vi "Query Client for Token.vi"(8 "error in (no error)":errorcluster, 10 "Request URI":string, 11 "OAuthClient in":refnum<class "OAuthClient.lvclass">) -> (0 "error out":errorcluster, 1 "Body":string, 2 "Header":string, 3 "OAuthClient out":refnum<class "OAuthClient.lvclass">)   [LabVIEW 2013, in "OAuthClient.lvclass"]
uses:
  OAuthClient.lvclass
  OAuthClient.lvclass/OAuthClient.ctl
  <vilib>/httpClient/POSTBuffer.vi
  <vilib>/httpClient/LabVIEWHTTPClient.lvlib
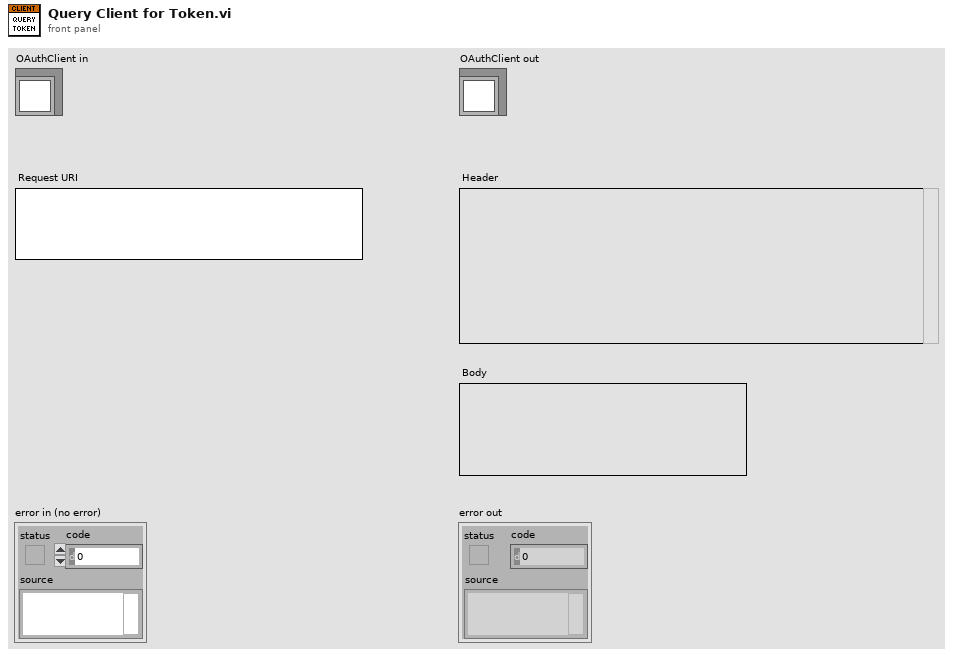
[diagram p1: front panel]
types:
  T1 = typedef "LabVIEWHTTPClient.lvlib/ClientHandle.ctl" = refnum<k1>
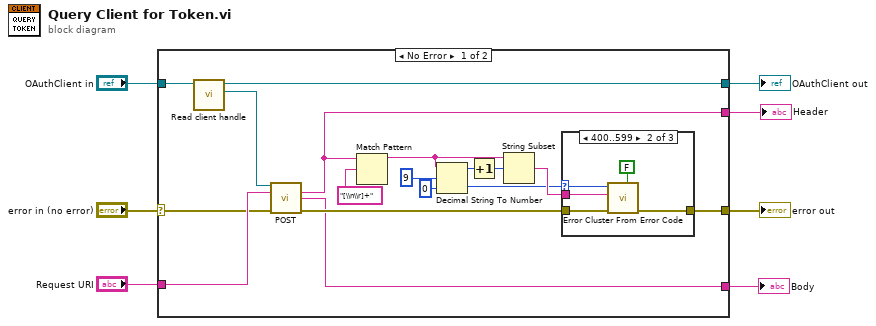
[diagram p0: block diagram]
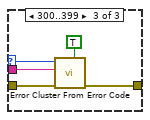
[diagram p3: hidden frame]
diagram:
  n1 = case shown="No Error" "error in (no error)" {
    selector: "error in (no error)" -> [w9 w37]
    tunnel: [w13 w37] -> w6
    tunnel: [w22 w36] -> w4
    tunnel: "OAuthClient in" -> [w24 w36]
    tunnel: "Request URI" -> [w23 _]
    tunnel: [w12 _] -> w2
    tunnel: [w10 _] -> w1
    frame No Error {
      n2 = call "Read client handle.vi"("OAuthClient in"=w24) -> ("Client Handle"=w8:T1, "OAuthClient out"=w22:refnum<class "OAuthClient.lvclass">)  [unwired: 8 in, 1 out]
      n3 = call-poly <vilib>:"POST.vi"("client handle"=w8, "url"=w23, "error in (no error)"=w9) -> ("headers"=w10:string, "body"=w12:string, "error out"=w14:errorcluster)  [unwired: 9 in, 1 out]
      n4 = Match Pattern(string=w10, regular expression="[\\n\\r]+") -> (before substring=w20:string)  [unwired: 1 in, 3 out]
      n5 = Decimal String To Number(string=w20, offset=u32 9 ("initial scan location"), default (0L)=0 ("default value 1")) -> (offset past number=w18:i32, number=w17:i32)
      n6 = Increment(x=w18) -> (x+1=w21:i32)
      n7 = String Subset(string=w20, offset (0)=w21) -> (substring=w19:string)  [unwired: 1 in]
      n8 = case shown="400..599" w17 {
        selector: w17 -> [_ w28 w33]
        tunnel: w14 -> [w25 w30 w35]
        tunnel: [w25 w29 w34] -> w13
        tunnel: w19 -> [_ w27 w32]
        frame Default {
        }
        frame 400..599 {
          n9 = call <vilib>:"Error Cluster From Error Code.vi"("is warning? (False)"=FALSE, "error in (no error)"=w30, "error message (\"\")"=w27, "error code (0)"=w28) -> ("error out"=w29:errorcluster)  [unwired: 5 in]
        }
        frame 300..399 {
          n10 = call <vilib>:"Error Cluster From Error Code.vi"("is warning? (False)"=TRUE, "error in (no error)"=w35, "error message (\"\")"=w32, "error code (0)"=w33) -> ("error out"=w34:errorcluster)  [unwired: 5 in]
        }
      }
    }
    frame Error {
    }
  }
  "error out" <- w6
  "OAuthClient out" <- w4
  "Body" <- w2
  "Header" <- w1
